vi "_077.vi"() -> ()   [LabVIEW 2024]
panel:
  out "Numeric 2":i32
  out "Array 7":i32[][](array[numeric])
  out "Array 6":i32[](array[numeric])
  out "Array 4":i32[](array[numeric])
  out "Array 5":i32[][](array[numeric])
  out "Array 3":i32[](array[numeric])
  out "Numeric":i32
  out "Array 2":i32[](array[numeric])
  out "Array":i32[](array[numeric])
  # "Fundamentals :"
  # "6~>After running this VI,what is the value displayed in the o/p ?"
  # "Nrml Approach :"
  # "Dfrnt Approach :"
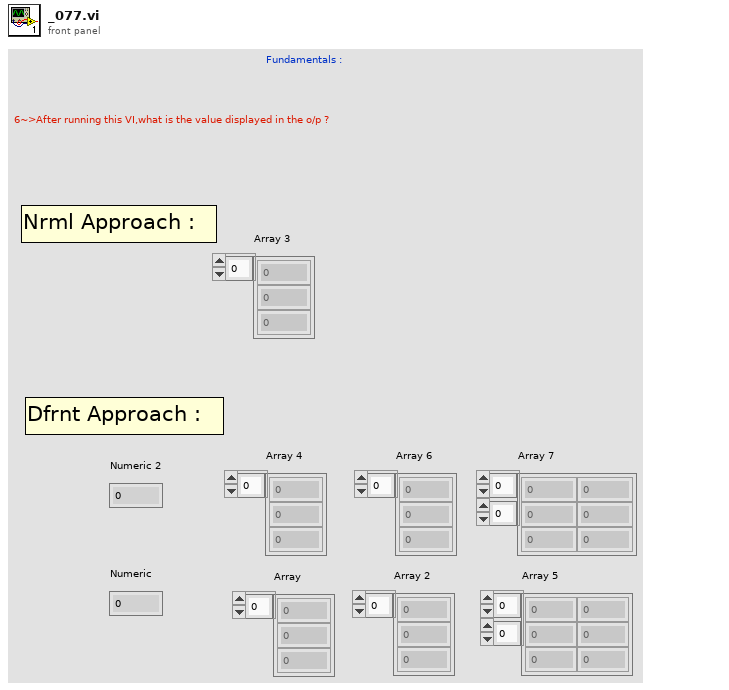
[diagram p1: front panel]
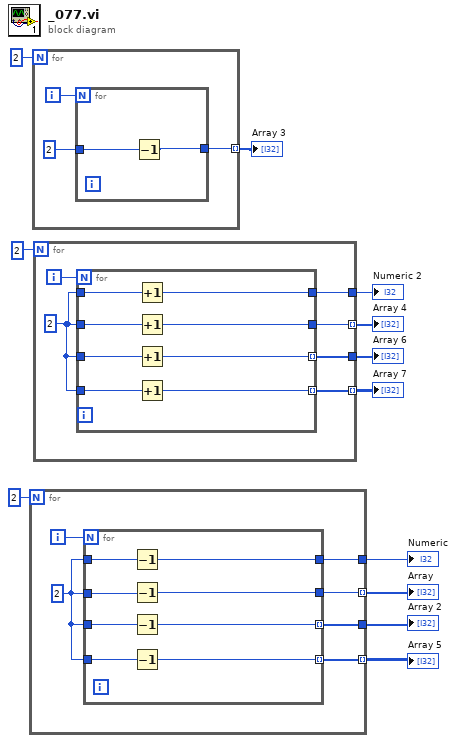
[diagram p0: block diagram]
diagram:
  n1 = for {
    N: 2 -> [_]
    tunnel: [w17] -> w11 mode=indexing
    tunnel: [w16] -> w10
    tunnel: [w15] -> w9
    tunnel: [w13] -> w6 mode=indexing
    i -> [w18]
    w14 = 2
    n2 = for {
      N: w18 -> [_]
      tunnel: w14 -> [w26]
      tunnel: [w25] -> w17
      tunnel: w14 -> [w24]
      tunnel: [w23] -> w16 mode=indexing
      tunnel: w14 -> [w22]
      tunnel: [w21] -> w15
      tunnel: w14 -> [w20]
      tunnel: [w19] -> w13 mode=indexing
      n3 = Decrement(x=w22) -> (x-1=w21:i32)
      n4 = Decrement(x=w26) -> (x-1=w25:i32)
      n5 = Decrement(x=w24) -> (x-1=w23:i32)
      n6 = Decrement(x=w20) -> (x-1=w19:i32)
    }
  }
  "Array" <- w11
  "Array 2" <- w10
  "Numeric" <- w9
  "Array 5" <- w6
  n7 = for {
    N: 2 -> [_]
    tunnel: [w28] -> w8 mode=indexing
    i -> [w29]
    n8 = for {
      N: w29 -> [_]
      tunnel: 2 -> [w31]
      tunnel: [w30] -> w28
      n9 = Decrement(x=w31) -> (x-1=w30:i32)
    }
  }
  "Array 3" <- w8
  n10 = for {
    N: 2 -> [_]
    tunnel: [w36] -> w4 mode=indexing
    tunnel: [w35] -> w3
    tunnel: [w34] -> w2 mode=indexing
    tunnel: [w32] -> w1
    i -> [w37]
    w33 = 2
    n11 = for {
      N: w37 -> [_]
      tunnel: w33 -> [w45]
      tunnel: [w44] -> w36
      tunnel: w33 -> [w43]
      tunnel: [w42] -> w35 mode=indexing
      tunnel: w33 -> [w41]
      tunnel: [w40] -> w34 mode=indexing
      tunnel: w33 -> [w39]
      tunnel: [w38] -> w32
      n12 = Increment(x=w39) -> (x+1=w38:i32)
      n13 = Increment(x=w45) -> (x+1=w44:i32)
      n14 = Increment(x=w43) -> (x+1=w42:i32)
      n15 = Increment(x=w41) -> (x+1=w40:i32)
    }
  }
  "Array 4" <- w4
  "Array 6" <- w3
  "Array 7" <- w2
  "Numeric 2" <- w1
